vi "Create.vi"(8 "error in (no error)":errorcluster, 10 "messageID":u16) -> (0 "error out":errorcluster, 3 "mqttCmdPublishAck out":refnum<class "PublishAckMqttMsg.lvclass">)   [LabVIEW 2020, in "PublishAckMqttMsg.lvclass"]
uses:
  PublishAckMqttMsg.lvclass
  PublishAckMqttMsg.lvclass/PublishAckMqttMsg.ctl
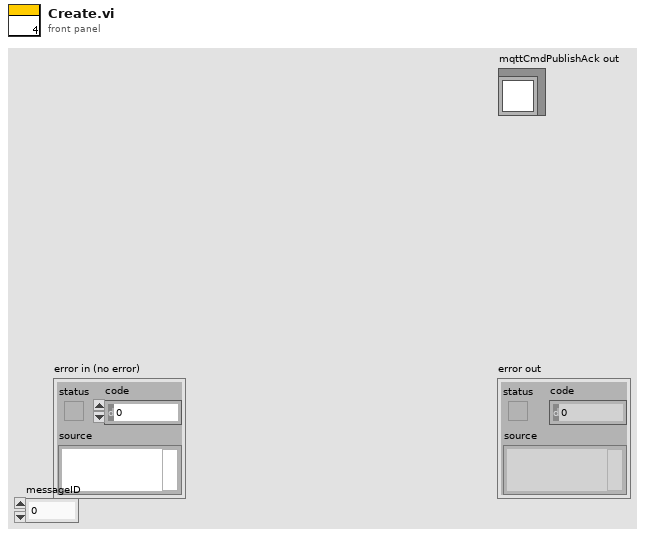
[diagram p1: front panel]
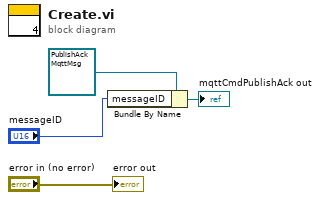
[diagram p0: block diagram]
diagram:
  n1 = Bundle By Name(cluster=refnum<class "PublishAckMqttMsg.lvclass"> refnum ("mqttCmdPublishAck in"), "messageID"="messageID") -> (→"mqttCmdPublishAck out":refnum<class "PublishAckMqttMsg.lvclass">)
  "error out" <- "error in (no error)"
